vi "get_SPEEDs.vi"(8 "error in (no error)":errorcluster caption="错误输入（无错误）", 11 "MotorSystem 输入":refnum<class "MotorSystem.lvclass">) -> (0 "error out":errorcluster caption="错误输出", 2 "speeds":i32[](array[numeric]), 3 "MotorSystem 输出":refnum<class "MotorSystem.lvclass">)   [LabVIEW 2016, in "MotionControl.lvlib" / "MotorSystem.lvclass"]
uses:
  <userlib>/MotionControl/MotorSystem/MotorSystem.lvclass
  <userlib>/MotionControl/MotorSystem/MotorSystem.lvclass/MotorSystem.ctl
  <userlib>/MotionControl/OneMotion/OneMotion.lvclass
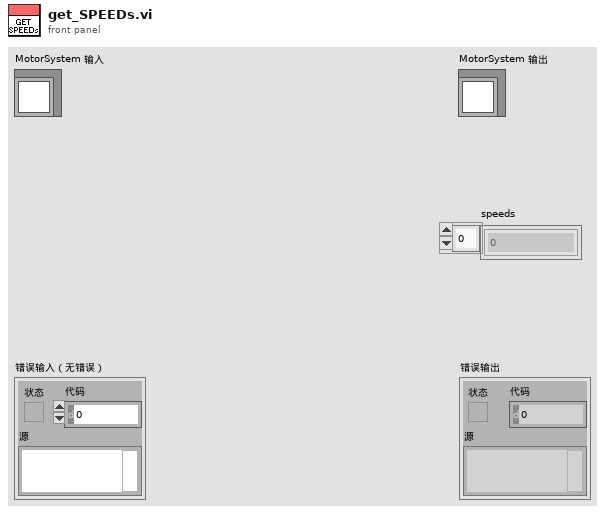
[diagram p1: front panel]
types:
  T1 = typedef "MotionControl.lvlib/MotorSystem.lvclass/MotionCluster.ctl" = cluster{"OneMotion.lvclass":refnum<class "OneMotion.lvclass">, "connected?":bool, "default enabled?":bool, "enabled?":bool}
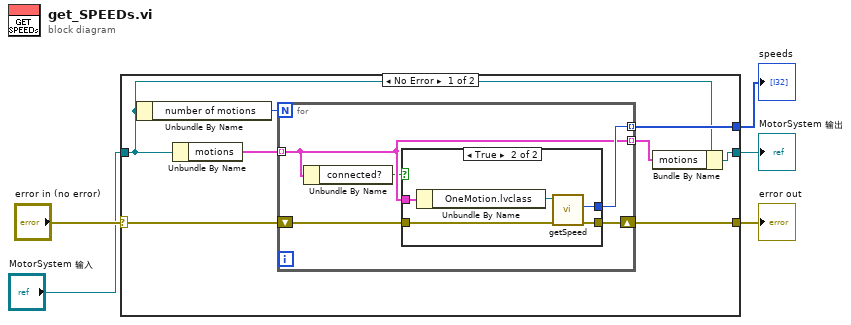
[diagram p0: block diagram]
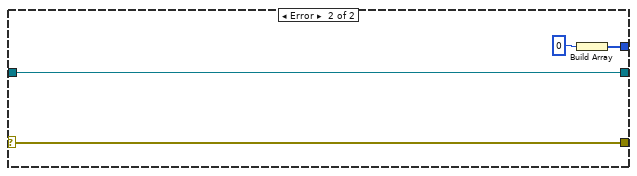
[diagram p3: hidden frame]
diagram:
  n1 = case shown="No Error" "error in (no error)" {
    selector: "error in (no error)" -> [w10 w28]
    tunnel: [w9 w28] -> w4
    tunnel: [w6 w27] -> w2
    tunnel: "MotorSystem 输入" -> [w8 w27]
    tunnel: [w11 w25] -> w1
    frame No Error {
      n2 = Unbundle By Name(w8) -> ("number of motions"=w13:i32)
      n3 = Unbundle By Name(w8) -> ("motions"=w12:T1[])
      n4 = for {
        N: w13 -> [_]
        tunnel: w12 -> [w15] mode=indexing
        tunnel: [w16] -> w11 mode=indexing
        shift-right: [w17] -> w9
        shift-left: w10 -> [w18]
        tunnel: [w15] -> w7 mode=indexing
        n5 = Unbundle By Name(w15) -> ("connected?"=w14:bool)
        n6 = case shown="True" w14 {
          tunnel: w18 -> [w19 w23]
          tunnel: [w19 w22] -> w17
          tunnel: [_ w21] -> w16
          tunnel: w15 -> [_ w20]
          frame False {
          }
          frame True {
            n7 = Unbundle By Name(w20) -> ("OneMotion.lvclass"=w24:refnum<class "OneMotion.lvclass">)
            n8 = call <userlib>:"getSpeed.vi"("error in (no error)"=w23, "OneMotion 输入"=w24) -> ("error out"=w22:errorcluster, "speed"=w21:i32)  [unwired: 7 in, 1 out]
          }
        }
      }
      n9 = Bundle By Name(cluster=w8, "motions"=w7) -> (w6:refnum<class "MotorSystem.lvclass">)
    }
    frame Error {
      n10 = Build Array(0) -> (w25:i32[])
    }
  }
  "error out" <- w4
  "MotorSystem 输出" <- w2
  "speeds" <- w1
